vi "Motor_Test.vi"() -> ()   [LabVIEW 2009]
uses:
  Controls/MotorStatus.ctl
panel:
  in  "<":bool
  in  ">":bool
  in  "StepSize":i32(slide) scale=0.0..100.0
  in  "Home":bool
  in  "Named":string
  out "Axis status":T1
  in  "stop":bool
  in  "MOTOR":string
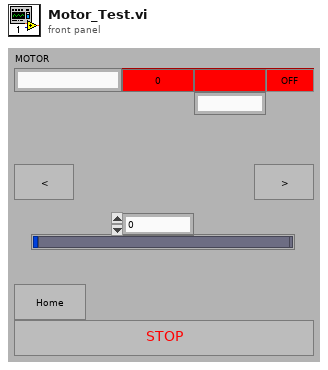
[diagram p1: front panel]
types:
  T1 = typedef "MotorStatus.ctl" = cluster{"Managed?":bool, "Position":i32, "Name":string, "Status":enum16{"OFF", "IDLE", "MOVING", "HOMING"}}
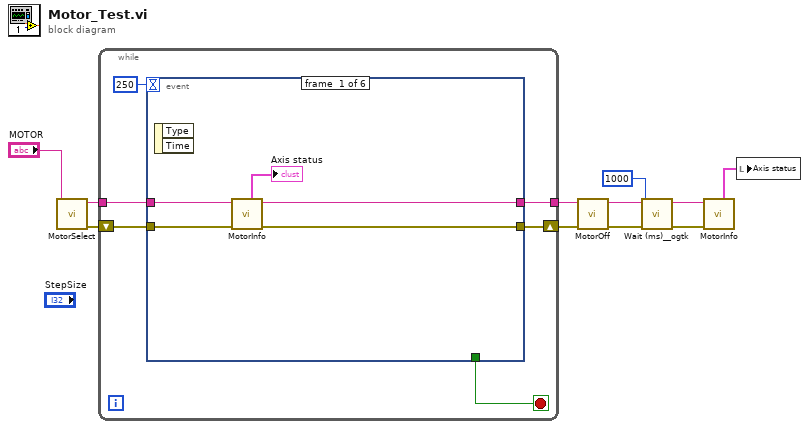
[diagram p0: block diagram]
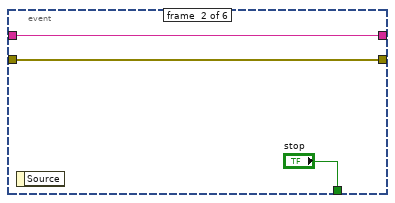
[diagram p2: hidden frame]
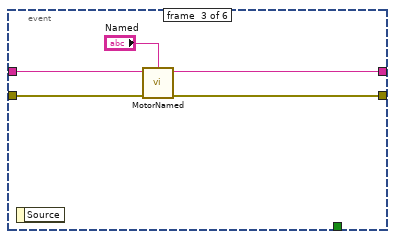
[diagram p3: hidden frame]
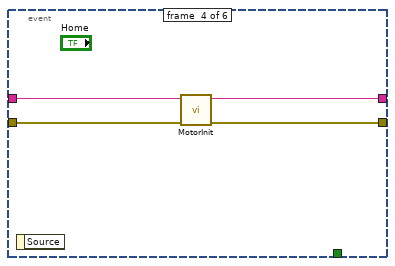
[diagram p4: hidden frame]
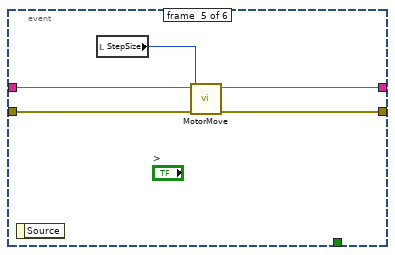
[diagram p5: hidden frame]
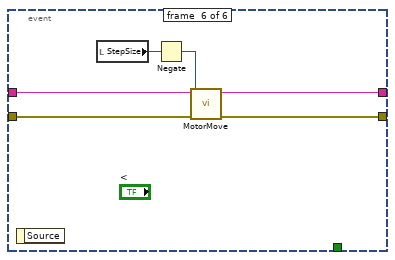
[diagram p6: hidden frame]
diagram:
  n1 = call "MotorSelect.vi"("Motor"="MOTOR") -> ("Motor out"=w9:string, "error out"=w8:errorcluster)  [unwired: 1 in, 6 out]
  n2 = while {
    shift-right: [w12] -> w7
    shift-left: w8 -> [w16]
    tunnel: w9 -> [w15]
    tunnel: [w13] -> w6
    stop <- w11 stop-if-true
    n3 = event shown="[5] \"<\": Value Change" {
      selector: _ -> [_ _ _ _ _ _]
      dyn-events: _ -> [_ _ _ _ _ _]
      timeout: 250 -> [_ _ _ _ _ _]
      tunnel: w16 -> [w21 w23 w29 w33 w38 w44]
      tunnel: w15 -> [w20 w22 w28 w31 w36 w42]
      tunnel: [w18 w22 w26 w30 w35 w41] -> w13
      tunnel: [w17 w23 w25 w32 w37 w43] -> w12
      tunnel: [_ "stop" _ _ _ _] -> w11
      event #0 {
        n4 = event-data() -> ()  [unwired: 3 out]
        n5 = call "MotorInfo.vi"("error in (no error)"=w21, "Motor"=w20) -> ("error out"=w17:errorcluster, "Motor out"=w18:string, "Axis status"=→"Axis status":T1)  [unwired: 5 out]
      }
      event #1 {
        n6 = event-data() -> ()  [unwired: 2 out]
      }
      event #2 {
        n7 = event-data() -> ()  [unwired: 2 out]
        n8 = call "MotorNamed.vi"("Name"="Named", "Motor in"=w28, "error in (no error)"=w29) -> ("Motor out"=w26:string, "error out"=w25:errorcluster)  [unwired: 5 out]
      }
      event #3 {
        n9 = event-data() -> ()  [unwired: 2 out]
        n10 = call "MotorInit.vi"("Motor"=w31, "error in (no error)"=w33) -> ("Motor out"=w30:string, "error out"=w32:errorcluster)  [unwired: 6 out]
      }
      event #4 {
        n11 = event-data() -> ()  [unwired: 2 out]
        n12 = local read "StepSize"() -> (w34:i32)
        n13 = call "MotorMove.vi"("Motor"=w36, "Movement"=w34, "error in (no error)"=w38) -> ("Motor out"=w35:string, "error out"=w37:errorcluster)  [unwired: 5 out]
      }
      event #5 {
        n14 = event-data() -> ()  [unwired: 2 out]
        n15 = local read "StepSize"() -> (w40:i32)
        n16 = Negate(x=w40) -> (-x=w39:i32)
        n17 = call "MotorMove.vi"("Motor"=w42, "Movement"=w39, "error in (no error)"=w44) -> ("Motor out"=w41:string, "error out"=w43:errorcluster)  [unwired: 5 out]
      }
    }
  }
  n18 = call "MotorOff.vi"("Motor"=w6, "error in (no error)"=w7) -> ("Motor out"=w5:string, "error out"=w3:errorcluster)  [unwired: 6 out]
  n19 = call <userlib>:"Wait (ms)__ogtk.vi"("error in (no error)"=w3, "milliseconds to wait"=u32 1000) -> ("error out"=w2:errorcluster)  [unwired: 1 in, 8 out]
  n20 = call "MotorInfo.vi"("error in (no error)"=w2, "Motor"=w5) -> ("Axis status"=w4:T1)  [unwired: 7 out]
  n21 = local write "Axis status"(w4) -> ()
